vi "CSM - Write INI String.vi"(5 "Section Name(\"\" as Default)":string, 7 "error in (no error)":errorcluster, 8 "String":string, 9 ">> Variable Name >>":string) -> (1 "error out":errorcluster, 2 "Key Replace?":bool)   [LabVIEW 2017, in "INI-Static-Variable-Support.lvlib"]
uses:
  INI-Static-Variable-Support.lvlib
  _fgv-oper.ctl
  <userlib>/_NEVSTOP/Communicable State Machine(CSM)/_Support/ChangeFlag/ChangeFlag-Read.vi
  <userlib>/_NEVSTOP/Communicable State Machine(CSM)/_Support/ChangeFlag/ChangeFlagDB.vi
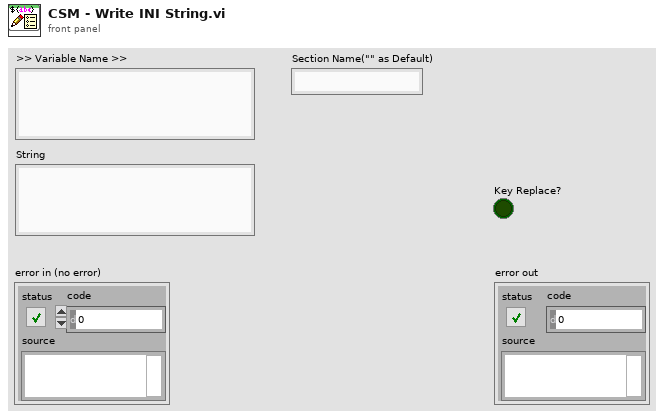
[diagram p1: front panel]
types:
  T1 = typedef "INI-Static-Variable-Support.lvlib/_fgv-oper.ctl" = enum16{"Read", "Write", "Sync", "Sessions", "List Keys", "Load", "List Files", "List Variables", "List Permanent Variables", "Mark Temp Variable as Permenent", "unload", "INIConfig(Memory)", "Reset", "Restore Variable Value"}
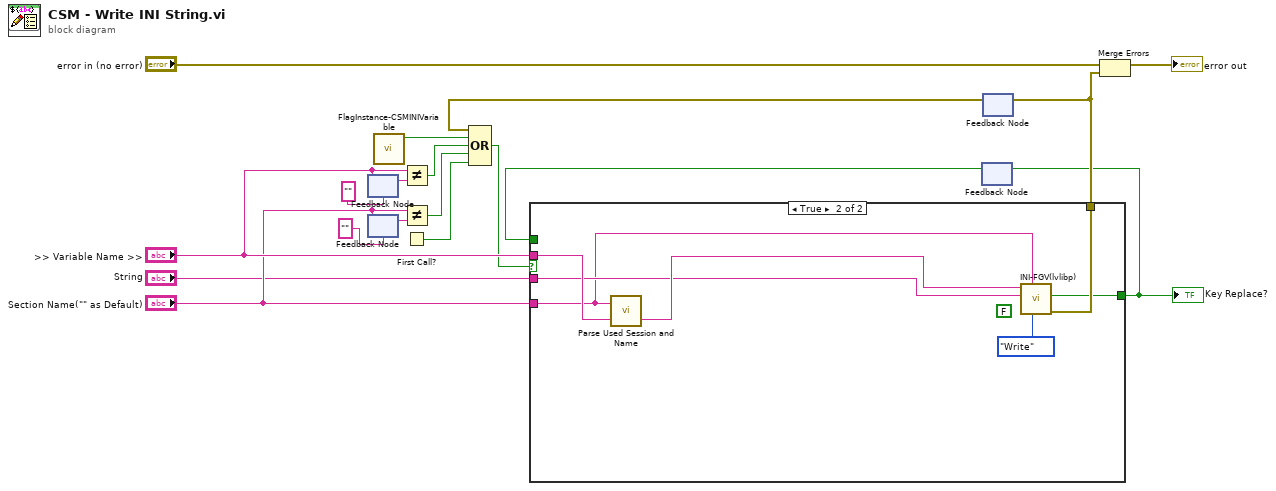
[diagram p0: block diagram]
diagram:
  n1 = feedback #1("") -> (w16:string)
  n2 = feedback-in #1(">> Variable Name >>") -> ()
  n3 = feedback #2("") -> (w15:string)
  n4 = feedback-in #2("Section Name(\"\" as Default)") -> ()
  n5 = call "FlagInstance-CSMINIVariable.vi"() -> ("Changed"=w1:bool)  [unwired: 10 in, 1 out]
  n6 = Not Equal?(x=">> Variable Name >>", y=w16) -> (x != y?=w12:bool)
  n7 = Not Equal?(x="Section Name(\"\" as Default)", y=w15) -> (x != y?=w11:bool)
  n8 = First Call?() -> (First Call?: T/F=w2:bool)
  n9 = feedback #3() -> (w8:bool)  [unwired: 1 in]
  n10 = feedback #4() -> (w7:errorcluster)  [unwired: 1 in]
  n11 = Compound Arithmetic op=OR(w7, w1, w12, w11, w2) -> (w6:bool)
  n12 = case shown="True" w6 {
    tunnel: [_ w25] -> w10
    tunnel: [w19 w24] -> w9
    tunnel: ">> Variable Name >>" -> [_ w23]
    tunnel: "Section Name(\"\" as Default)" -> [_ w20]
    tunnel: w8 -> [w19 _]
    tunnel: "String" -> [_ w21]
    frame False {
    }
    frame True {
      (unwired) FALSE ("Raw String? (F)")
      n13 = call "Parse Used Session and Name.vi"("name"=w23, "Section Name(\"\" as Default)"=w20) -> ("used name"=w22:string)  [unwired: 1 in]
      n14 = call "INI-FGV(lvlibp).vi"("Enum"=_fgv-oper."Write", "Prefered Section"=w20, ">> Default Value >>"=w21, ">> Variable Name >>"=w22) -> ("error out"=w25:errorcluster, "Key?"=w24:bool)  [unwired: 4 in, 2 out]
    }
  }
  "Key Replace?" <- w9
  n15 = feedback-in #3(w9) -> ()
  n16 = feedback-in #4(w10) -> ()
  n17 = Merge Errors("error in (no error)", w10) -> (→"error out":errorcluster)
